vi "Run Custom Device Pre Initialization VI.vi"(8 "error in (no error)":errorcluster, 10 "Settings":T2(array[cluster]), 11 "Pre Initialization VI":path) -> (0 "error out":errorcluster, 3 "Custom Device Ref":T1)   [LabVIEW 2019, in "Simple SysDef API.lvlib"]
uses:
  <userlib>/SimpleSysDef/Simple SysDef API.lvlib
  <userlib>/SimpleSysDef/_SubVIs/Custom Device Control Name and Ref.ctl
  NationalInstruments.VeriStand.SystemDefinitionAPI
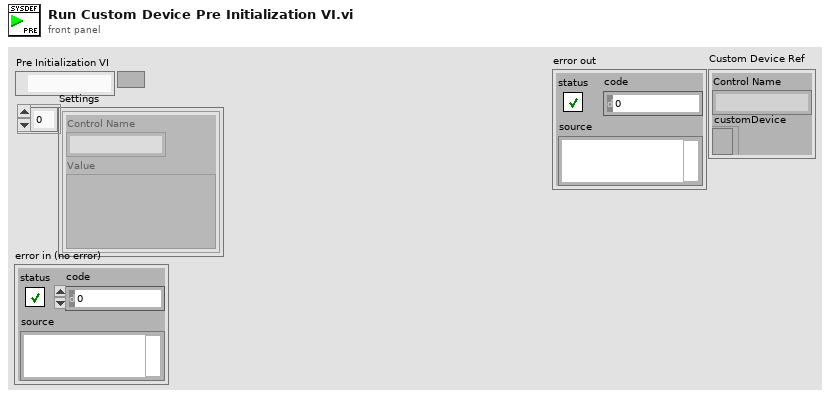
[diagram p1: front panel]
types:
  T1 = typedef "Simple SysDef API.lvlib/Custom Device Control Name and Ref.ctl" = cluster{"customDevice":refnum<k24>, "Control Name":string}
  T2 = cluster{"Control Name":string, "Value":variant}[]
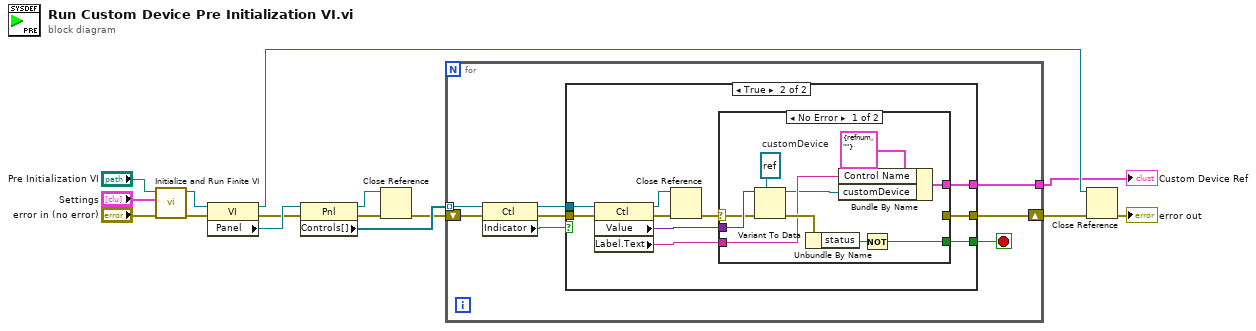
[diagram p0: block diagram]
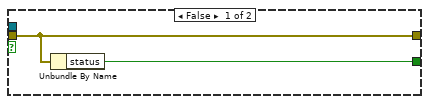
[diagram p2: hidden frame]
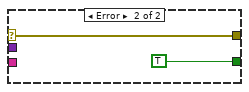
[diagram p3: hidden frame]
diagram:
  n1 = call <userlib>:"Initialize and Run Finite VI.vi"("error in (no error)"="error in (no error)", "Settings"="Settings", "Initialization VI"="Pre Initialization VI") -> ("error out"=w14:errorcluster, "VI out"=w13:refnum<vi>)  [unwired: 7 in]
  n2 = property class="VI"(reference=w13, error in=w14) -> (reference out=w12:refnum<vi>, error out=w10:errorcluster, "Panel"=w11:refnum<vi>)
  n3 = property class="Pnl"(reference=w11, error in=w10) -> (reference out=w8:refnum<vi>, error out=w9:errorcluster, "Controls[]"=w7:refnum<vi>[])
  n4 = Close Reference(reference=w8, error in (no error)=w9) -> (error out=w6:errorcluster)
  n5 = for {
    tunnel: w7 -> [w23] mode=indexing
    shift-right: [w18] -> w5
    shift-left: w6 -> [w22]
    tunnel: [w17] -> w1
    stop <- w16 stop-if-true
    n6 = property class="Ctl"(reference=w23, error in=w22) -> (reference out=w19:refnum<vi>, error out=w20:errorcluster, "Indicator"=w21:bool)
    n7 = case shown="True" w21 {
      tunnel: w20 -> [w25 w35]
      tunnel: w19 -> [_ w34]
      tunnel: [w25 w28] -> w18
      tunnel: [w24 w29] -> w16
      tunnel: [_ w27] -> w17
      frame False {
        n8 = Unbundle By Name(w25) -> ("status"=w24:bool)
      }
      frame True {
        n9 = property class="Ctl"(reference=w34, error in=w35) -> (reference out=w31:refnum<vi>, error out=w32:errorcluster, "Value"=w33:variant, "Label.Text"=w26:string)
        n10 = Close Reference(reference=w31, error in (no error)=w32) -> (error out=w30:errorcluster)
        n11 = case shown="No Error" w30 {
          selector: w30 -> [w42 w47]
          tunnel: w33 -> [w45 _]
          tunnel: [w40 TRUE] -> w29
          tunnel: [_ w47] -> w28
          tunnel: [w37 _] -> w27
          tunnel: w26 -> [w39 _]
          frame No Error {
            w44 = refnum<k24> refnum  # customDevice
            n12 = Variant To Data(error in=w42, type=w44, Variant=w45) -> (data=w38:refnum<k24>, error out=w43:errorcluster)
            n13 = Unbundle By Name(w43) -> ("status"=w41:bool)
            n14 = Bundle By Name(cluster=T1 {"customDevice"=refnum, "Control Name"=""} ("Custom Device Ref"), "Control Name"=w39, "customDevice"=w38) -> (w37:T1)
            n15 = Not(x=w41) -> (.not. x?=w40:bool)
          }
          frame Error {
          }
        }
      }
    }
  }
  "Custom Device Ref" <- w1
  n16 = Close Reference(reference=w12, error in (no error)=w5) -> (error out=→"error out":errorcluster)
